vi "LED States to Word.vi"(11 "LED States":T1) -> (3 "LED Word":u16)   [LabVIEW 2014, in "SLSC configuration Shared.lvlib"]
doc: "Converts four faults to a fault word."
uses:
  SLSC configuration Shared.lvlib
  Bank LED States.ctl
  LED State.ctl
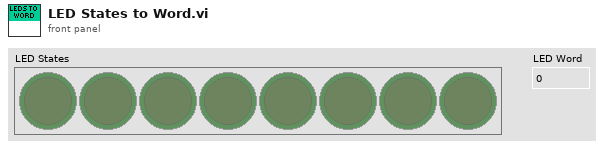
[diagram p1: front panel]
types:
  T1 = typedef "SLSC configuration Shared.lvlib/Bank LED States.ctl" = T2[]
  T2 = typedef "SLSC configuration Shared.lvlib/LED State.ctl" = bool
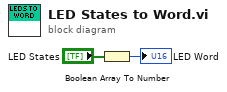
[diagram p0: block diagram]
diagram:
  n1 = Boolean Array To Number(Boolean array="LED States") -> (number=→"LED Word":u16)
